vi "ReadPath.vi"() -> (3 "Lanes":T1)   [LabVIEW 2013]
uses:
  <vilib>/imath/engines/lvmath2/RunTimeEngine/ErrorHandling/NIMS_Finalize Error.vi
  <vilib>/imath/engines/lvmath2/RunTimeEngine/IndexRead/NIMS M($,S).vi
  <instcachedir>/0/NIMS M($,S)_3E5749BBB62E49528D4765A77F1F6D98.lvgen/NIMS M($,S)_3E5749BBB62E49528D4765A77F1F6D98_000.vi
  <vilib>/imathl/engines/lvmath/Functions/Error Handling/Create Error.vi
  <vilib>/imath/engines/lvmath2/RunTimeEngine/NodeEndStatement/NIMS_NodeEndStatement_Output.vi
  <instcachedir>/0/NIMS_NodeEndStatement_Output_53EC0D466D134D7ABD903AC30B43404B.lvgen/NIMS_NodeEndStatement_Output_53EC0D466D134D7ABD903AC30B43404B_002.vi
  <vilib>/imath/engines/lvmath2/RunTimeEngine/BuiltInFunctions/difference/NIMS_difference(GV,I32).vi
  <instcachedir>/0/NIMS_difference(GV,I32)_DC7351DCBCF840A8AE147F50EC2CE86E.lvgen/NIMS_difference(GV,I32)_DC7351DCBCF840A8AE147F50EC2CE86E_000.vi
  <vilib>/imath/engines/lvmath2/RunTimeEngine/BuiltInFunctions/atan2/NIMS_atan2(A,A).vi
  <instcachedir>/0/NIMS_atan2(A,A)_2936FD7F864E46C682B467FE18724EF9.lvgen/NIMS_atan2(A,A)_2936FD7F864E46C682B467FE18724EF9_004.vi
  <vilib>/imath/engines/lvmath2/RunTimeEngine/IndexRead/NIMS V(S).vi
  <instcachedir>/0/NIMS V(S)_0488751826AF41519A22953C041130DC.lvgen/NIMS V(S)_0488751826AF41519A22953C041130DC_000.vi
  <vilib>/imath/engines/lvmath2/RunTimeEngine/RowToken/NIMS_RowToken_CV_CV.vi
  <instcachedir>/0/NIMS_RowToken_CV_CV_C399A8ED4CD3472C8B972CCEAF5D750A.lvgen/NIMS_RowToken_CV_CV_C399A8ED4CD3472C8B972CCEAF5D750A_000.vi
  <vilib>/imath/engines/lvmath2/RunTimeEngine/RowToken/NIMS_RowToken_M_CV.vi
  <instcachedir>/0/NIMS_RowToken_M_CV_4FFFB80A1A2C4A06BEF1E2564C6BAFA4.lvgen/NIMS_RowToken_M_CV_4FFFB80A1A2C4A06BEF1E2564C6BAFA4_000.vi
  <vilib>/imath/engines/lvmath2/RunTimeEngine/ErrorHandling/NIMS_Create Error From Enums.vi
types:
  T1 = cluster{"Right_lane":dbl[][], "Center_lane":dbl[][], "Left_lane":dbl[][]}
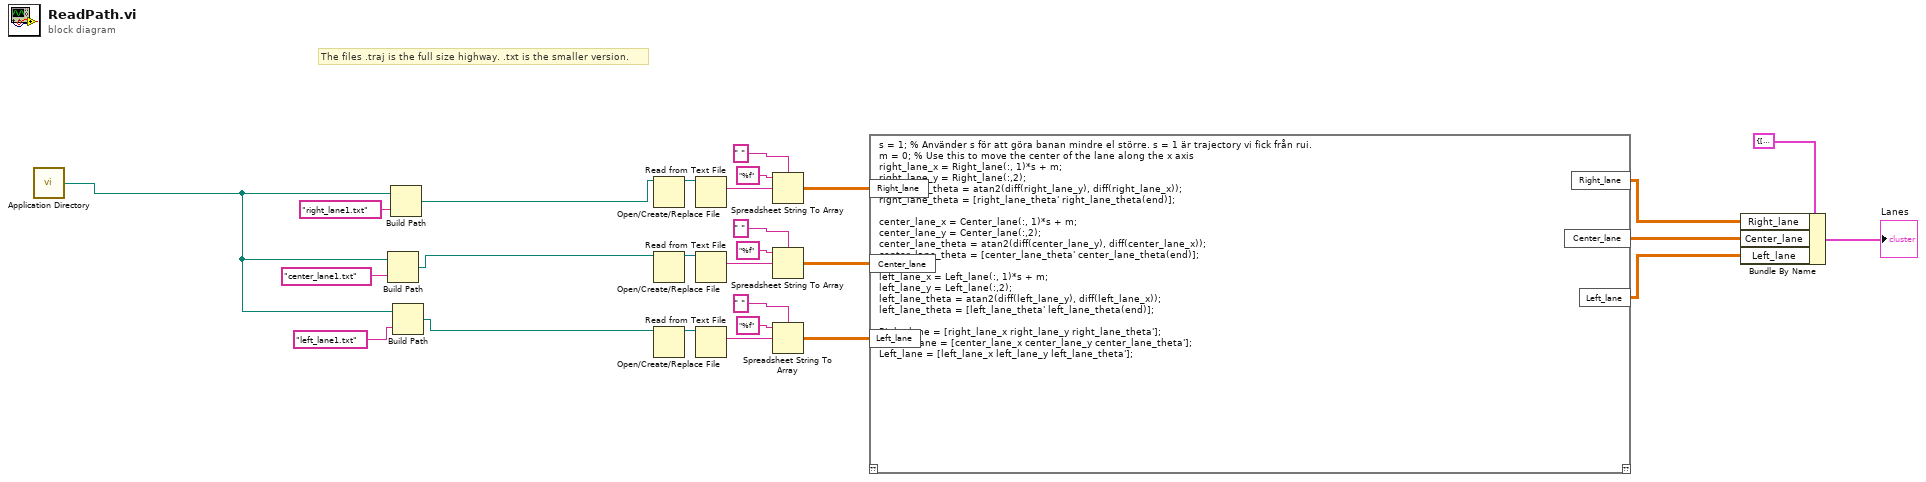
[diagram p0: block diagram]
diagram:
  # "The files .traj is the full size highway. .txt is the smaller version."
  n1 = call <vilib>:"Application Directory.vi"() -> ("Application Directory"=w1:path)
  n2 = Build Path(base path=w1, name or relative path="center_lane1.txt") -> (appended path=w3:path)
  n3 = Build Path(base path=w1, name or relative path="right_lane1.txt") -> (appended path=w6:path)
  n4 = Build Path(base path=w1, name or relative path="left_lane1.txt") -> (appended path=w2:path)
  n5 = Open/Create/Replace File(file path (use dialog)=w6) -> (refnum out=w27:refnum<file>)  [unwired: 5 in, 2 out]
  n6 = Open/Create/Replace File(file path (use dialog)=w3) -> (refnum out=w19:refnum<file>)  [unwired: 5 in, 2 out]
  n7 = Open/Create/Replace File(file path (use dialog)=w2) -> (refnum out=w23:refnum<file>)  [unwired: 5 in, 2 out]
  n8 = Read from Text File(file (use dialog)=w27) -> (text=w26:string)  [unwired: 3 in, 3 out]
  n9 = Read from Text File(file (use dialog)=w19) -> (text=w18:string)  [unwired: 3 in, 3 out]
  n10 = Read from Text File(file (use dialog)=w23) -> (text=w22:string)  [unwired: 3 in, 3 out]
  n11 = Spreadsheet String To Array(delimiter (Tab)=" ", format string="%f", spreadsheet string=w26) -> (array=w13:dbl[][])  [unwired: 1 in]
  n12 = Spreadsheet String To Array(delimiter (Tab)=" ", format string="%f", spreadsheet string=w18) -> (array=w15:dbl[][])  [unwired: 1 in]
  n13 = Spreadsheet String To Array(delimiter (Tab)=" ", format string="%f", spreadsheet string=w22) -> (array=w14:dbl[][])  [unwired: 1 in]
  n14 = mathscript code="s = 1; % Använder s för att göra banan mindre el större. s = 1 är trajectory vi fick från rui.\nm = 0; % Use this to move the center of the lane along the x axis\nright_lane_x = Right_lane(:, 1)*s + m;\nright_lane_y = Right_lane(:,2);\nright_lane_theta = atan2(diff(right_lane_y), diff(right_lane_x));\nright_lane_theta = [right_lane_theta' right_lane_theta(end)];\n\ncenter_lane_x = Center_lane(:, 1)*s + m;\ncenter_lane_y = Center_lane(:,2);\ncenter_lane_theta = atan2(diff(center_lane_y), diff(center_lane_x));\ncenter_lane_theta = [center_lane_theta' center_lane_theta(end)];\n\nleft_lane_x = Left_lane(:, 1)*s + m;\nleft_lane_y = Left_lane(:,2);\nleft_lane_theta = atan2(diff(left_lane_y), diff(left_lane_x));\nleft_lane_theta = [left_lane_theta' left_lane_theta(end)];\n\nRight_lane = [right_lane_x right_lane_y right_lane_theta'];\nCenter_lane = [center_lane_x center_lane_y center_lane_theta'];\nLeft_lane = [left_lane_x left_lane_y left_lane_theta'];"("Right_lane"=w13, "Left_lane"=w14, "Center_lane"=w15) -> ("Right_lane"=w10:dbl[][], "Center_lane"=w9:dbl[][], "Left_lane"=w8:dbl[][])  [unwired: 1 in, 1 out]
  n15 = Bundle By Name(cluster=T1 {"Right_lane"=[], "Center_lane"=[], "Left_lane"=[]} ("Lanes"), "Right_lane"=w10, "Center_lane"=w9, "Left_lane"=w8) -> (→"Lanes":T1)
